vi "FGV DRV stand.vi"(6 "Enum":enum16{"Write", "Read"}(ring)=enum."Read", 11 "DRV stand  in":T1) -> (3 "DRV stand out":T1)   [LabVIEW 2018, in "Application.lvlib"]
uses:
  Application.lvlib
  DRV stand.ctl
panel:
  in  "error in (no error)":errorcluster
  out "error out":errorcluster
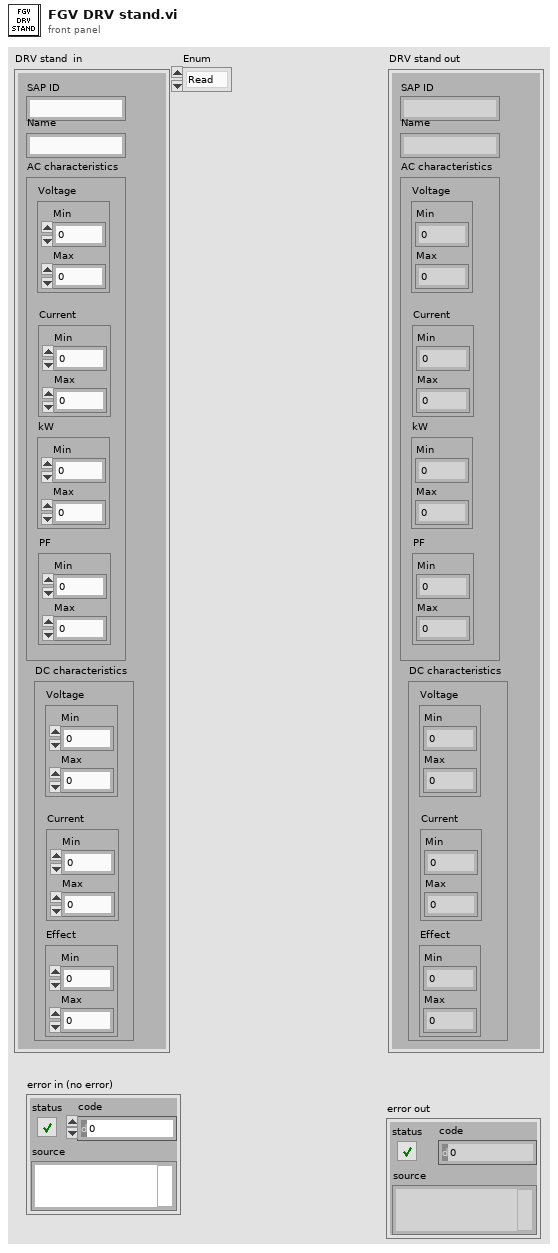
[diagram p1: front panel]
types:
  T1 = typedef "Application.lvlib/DRV stand.ctl" = cluster{"SAP ID":string, "Name":string, "AC characteristics":cluster{"Voltage":cluster{"Min":dbl, "Max":dbl}, "Current":cluster{"Min":dbl, "Max":dbl}, "kW":cluster{"Min":dbl, "Max":dbl}, "PF":cluster{"Min":dbl, "Max":dbl}}, "DC characteristics":cluster{"Voltage":cluster{"Min":dbl, "Max":dbl}, "Current":cluster{"Min":dbl, "Max":dbl}, "Effect":cluster{"Min":dbl, "Max":dbl}}}
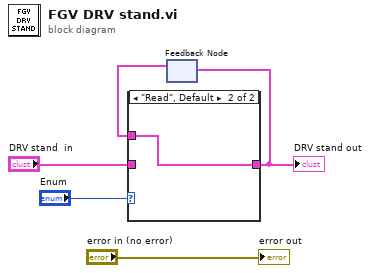
[diagram p0: block diagram]
diagram:
  n1 = feedback #1() -> (w3:T1)  [unwired: 1 in]
  n2 = case shown="\"Read\", Default" "Enum" {
    tunnel: "DRV stand  in" -> [w6 _]
    tunnel: [w6 w7] -> w2
    tunnel: w3 -> [_ w7]
    frame "Write" {
    }
    frame "Read", Default {
    }
  }
  "DRV stand out" <- w2
  n3 = feedback-in #1(w2) -> ()
  "error out" <- "error in (no error)"
